vi "U8ArrayToU16BigEndian(SubVI).vi"(10 "Numeric 7":u8 format="%x", 11 "Numeric 6":u8 format="%x") -> (3 "Numeric 9":u16 format="%x")   [LabVIEW 2012]
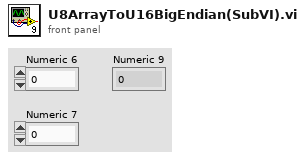
[diagram p1: front panel]
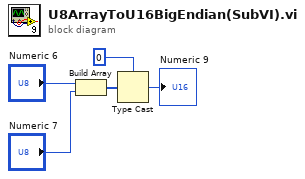
[diagram p0: block diagram]
diagram:
  n1 = Build Array("Numeric 6", "Numeric 7") -> (w3:u8[])
  n2 = Type Cast(type=u16 0, x=w3) -> (*(type *) &x=→"Numeric 9":u16)
